vi "Post-Install Custom Action.vi"(10 "Variant":variant) -> (0 "error out":errorcluster)   [LabVIEW 2020]
uses:
  <vilib>/zip/NI_Unzip.lvlib
  <vilib>/ErrorRing/Error Ring.xnode
  <vilib>/Utility/error.llb/Error Cluster From Error Code.vi
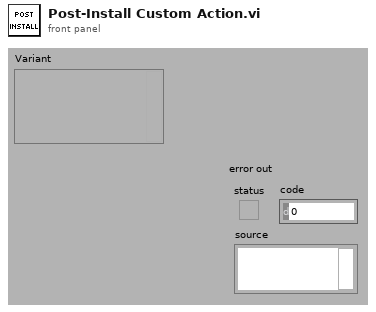
[diagram p1: front panel]
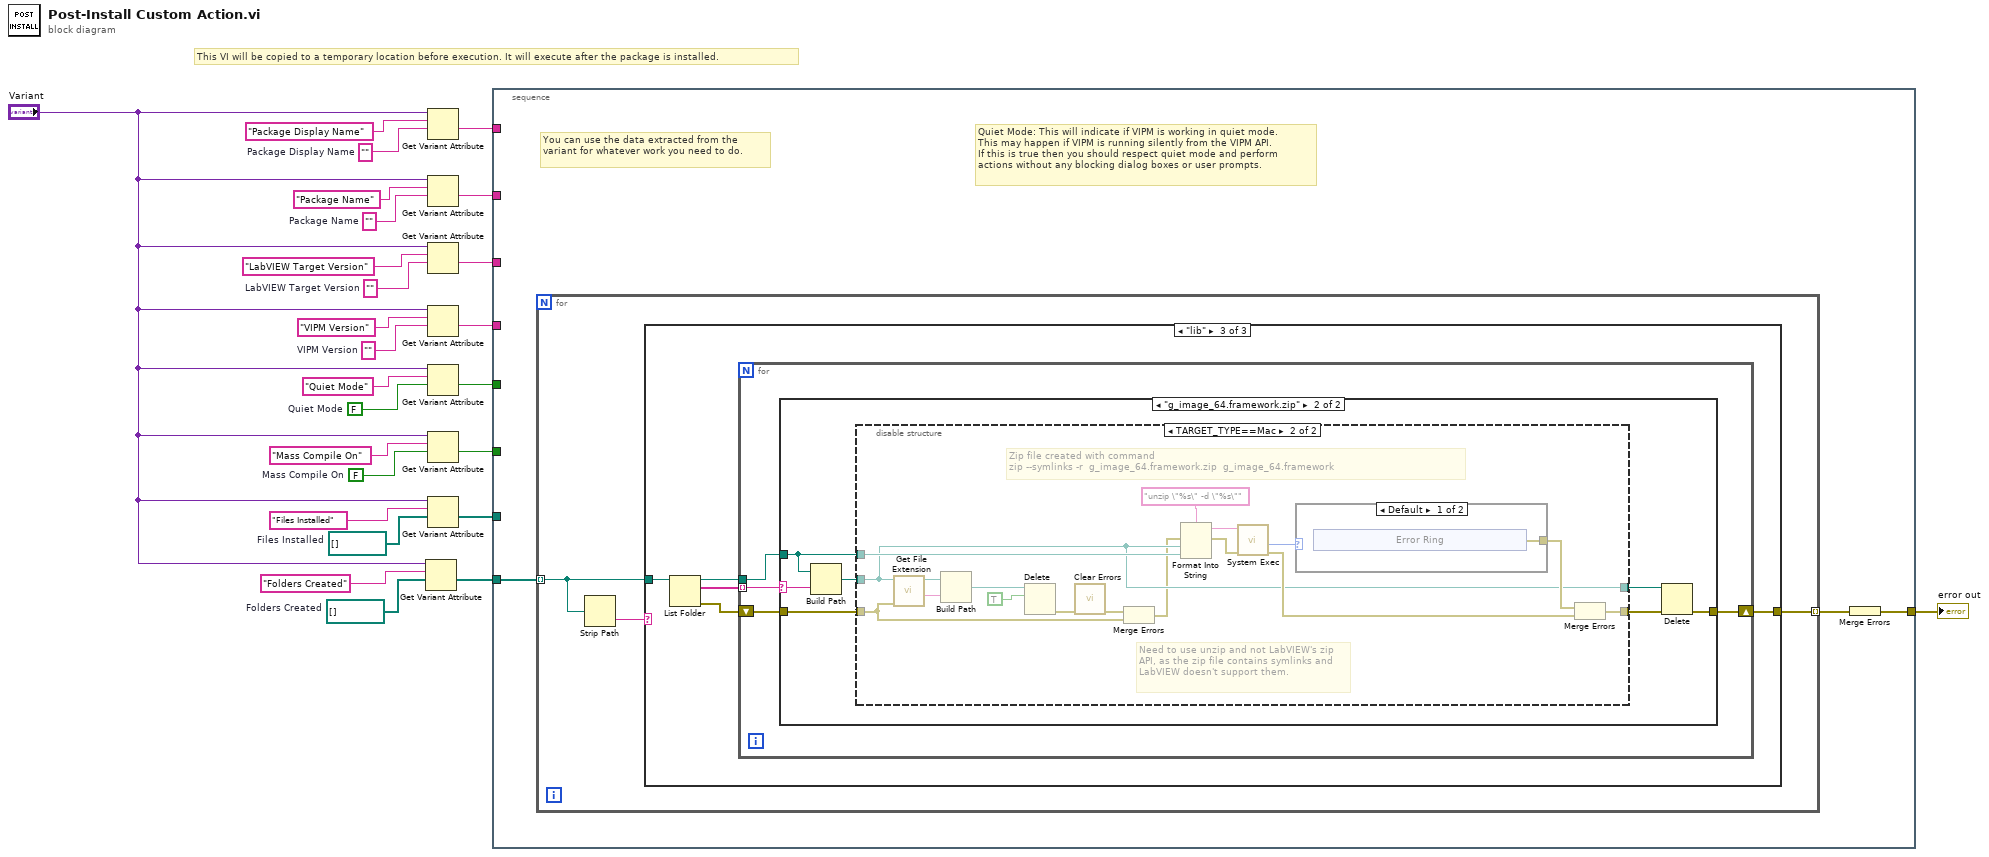
[diagram p0: block diagram]
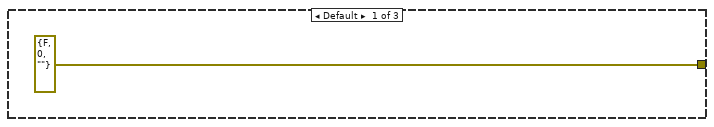
[diagram p2: hidden frame]
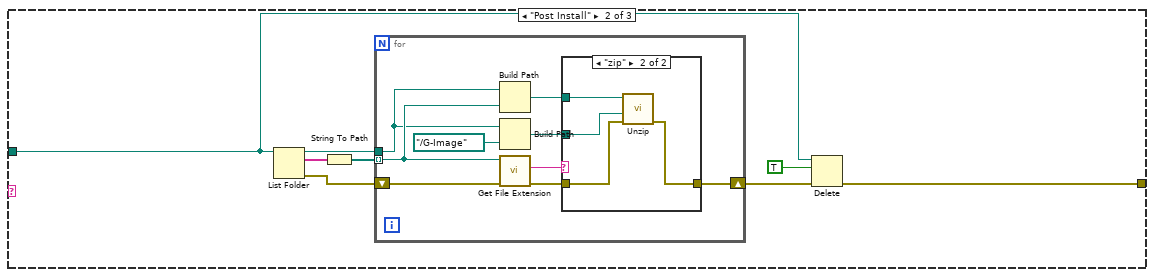
[diagram p3: hidden frame]
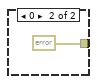
[diagram p7: hidden frame]
diagram:
  w2 = path[] []  # Folders Created
  w3 = path[] []  # Files Installed
  w9 = FALSE  # Mass Compile On
  w10 = ""  # Package Display Name
  w17 = FALSE  # Quiet Mode
  w20 = ""  # VIPM Version
  w22 = ""  # LabVIEW Target Version
  w24 = ""  # Package Name
  # "This VI will be copied to a temporary location before execution. It will execute after the package is installed."
  n1 = Get Variant Attribute(Variant="Variant", name="Folders Created", default value (empty Variant)=w2) -> (value=w7:path[])  [unwired: 1 in, 3 out]
  n2 = Get Variant Attribute(Variant="Variant", name="Package Display Name", default value (empty Variant)=w10) -> (value=w16:string)  [unwired: 1 in, 3 out]
  n3 = Get Variant Attribute(Variant="Variant", name="Package Name", default value (empty Variant)=w24) -> (value=w15:string)  [unwired: 1 in, 3 out]
  n4 = Get Variant Attribute(Variant="Variant", name="LabVIEW Target Version", default value (empty Variant)=w22) -> (value=w14:string)  [unwired: 1 in, 3 out]
  n5 = Get Variant Attribute(Variant="Variant", name="VIPM Version", default value (empty Variant)=w20) -> (value=w13:string)  [unwired: 1 in, 3 out]
  n6 = Get Variant Attribute(Variant="Variant", name="Quiet Mode", default value (empty Variant)=w17) -> (value=w12:bool)  [unwired: 1 in, 3 out]
  n7 = Get Variant Attribute(Variant="Variant", name="Mass Compile On", default value (empty Variant)=w9) -> (value=w11:bool)  [unwired: 1 in, 3 out]
  n8 = Get Variant Attribute(Variant="Variant", name="Files Installed", default value (empty Variant)=w3) -> (value=w6:path[])  [unwired: 1 in, 3 out]
  n9 = stacked-sequence {
    tunnel: w16 -> [_]
    tunnel: w15 -> [_]
    tunnel: w14 -> [_]
    tunnel: w13 -> [_]
    tunnel: w12 -> [_]
    tunnel: w11 -> [_]
    tunnel: w6 -> [_]
    tunnel: w7 -> [w29]
    tunnel: [w27] -> w1
    frame #0 {
      # "Quiet Mode: This will indicate if VIPM is working in quiet mode.\nThis may happen if VIPM is running silently from the VIPM API.\nIf this is true then you should respect quiet mode and perform\nactions without any blocking dialog boxes or user prompts."
      # "You can use the data extracted from the variant for whatever work you need to do."
      n10 = for {
        tunnel: w29 -> [w32] mode=indexing
        tunnel: [w31] -> w28 mode=indexing
        n11 = Strip Path(path=w32) -> (name=w30:string)  [unwired: 1 out]
        n12 = case shown="\"lib\"" w30 {
          tunnel: w32 -> [_ w35 w58]
          tunnel: [errorcluster {"status"=FALSE, "code"=0, "source"=""} ("error out") w36 w57] -> w31
          frame Default {
          }
          frame "Post Install" {
            n13 = List Folder(path=w35) -> (path out=w39:path, filenames=w41:string[], error out=w38:errorcluster)  [unwired: 3 in, 1 out]
            n14 = String To Path(string=w41) -> (path=w40:path[])
            n15 = for {
              tunnel: w40 -> [w50] mode=indexing
              tunnel: w39 -> [w43]
              shift-right: [w45] -> w37
              shift-left: w38 -> [w47]
              n16 = Build Path(base path=w43, name or relative path=w50) -> (appended path=w48:path)
              n17 = Build Path(base path=w43, name or relative path=path "../G-Image" ("Target directory (same as Zip file if empty)")) -> (appended path=w42:path)
              n18 = call <vilib>:"Get File Extension.vi"("error in (no error)"=w47, "file"=w50) -> ("error out"=w46:errorcluster, "lowercase file extension"=w49:string)  [unwired: 5 in, 3 out]
              n19 = case shown="\"zip\"" w49 {
                tunnel: w48 -> [_ w55]
                tunnel: w46 -> [w51 w54]
                tunnel: [w51 w53] -> w45
                tunnel: w42 -> [_ w52]
                frame Default {
                }
                frame "zip" {
                  n20 = call <vilib>:"Unzip.vi"("error in (no error)"=w54, "Target directory (same as Zip file if empty)"=w52, "Zip file"=w55) -> ("error out"=w53:errorcluster)  [unwired: 6 in, 2 out]
                }
              }
            }
            n21 = Delete(path (use dialog)=w35, entire hierarchy (F)=TRUE, error in=w37) -> (error out=w36:errorcluster)  [unwired: 2 in, 2 out]
          }
          frame "lib" {
            n22 = List Folder(path=w58) -> (path out=w60:path, filenames=w56:string[], error out=w59:errorcluster)  [unwired: 3 in, 1 out]
            n23 = for {
              tunnel: w60 -> [w61]
              shift-right: [w64] -> w57
              shift-left: w59 -> [w63]
              tunnel: w56 -> [w62] mode=indexing
              n24 = case shown="\"g_image_64.framework.zip\"" w62 {
                selector: w62 -> [_ w72]
                tunnel: w63 -> [w65 w70]
                tunnel: [w65 w68] -> w64
                tunnel: w61 -> [_ w67]
                frame Default {
                }
                frame "g_image_64.framework.zip" {
                  n25 = Build Path(base path=w67, name or relative path=w72) -> (appended path=w71:path)
                  n26 = disable-structure shown="TARGET_TYPE==Mac" {
                    disable-tunnel: w71 -> [w73 w81]
                    disable-tunnel: w67 -> [_ w89]
                    disable-tunnel: w70 -> [w74 w77]
                    disable-tunnel: [w74 w87] -> w69
                    disable-tunnel: [w73 w81] -> w66
                    frame condition #0 (active) {
                    }
                    frame condition #1 {
                      # "Zip file created with command\nzip --symlinks -r  g_image_64.framework.zip  g_image_64.framework"
                      # "Need to use unzip and not LabVIEW's zip API, as the zip file contains symlinks and LabVIEW doesn't support them."
                      n27 = call <vilib>:"Get File Extension.vi"("error in (no error)"=w77, "file"=w81) -> ("filename without extension"=w82:string, "dup file"=w79:path)  [unwired: 5 in, 3 out]
                      n28 = Build Path(base path=w79, name or relative path=w82) -> (appended path=w80:path)
                      n29 = Delete(path (use dialog)=w80, entire hierarchy (F)=TRUE) -> (error out=w78:errorcluster)  [unwired: 3 in, 2 out]
                      n30 = call <vilib>:"Clear Errors.vi"("error in (no error)"=w78) -> ("error out"=w76:errorcluster)  [unwired: 5 in, 1 out]
                      n31 = Merge Errors(w76, w77) -> (w75:errorcluster)
                      n32 = Format Into String(format string="unzip \"%s\" -d \"%s\"" ("command line"), error in=w75, w81, w89) -> (resulting string=w86:string, error out=w90:errorcluster)  [unwired: 1 in]
                      n33 = call <vilib>:"System Exec.vi"("error in (no error)"=w90, "command line"=w86) -> ("error out"=w84:errorcluster, "return code"=w85:i32)  [unwired: 6 in, 2 out]
                      n34 = case shown="Default" w85 {
                        tunnel: [w92 errorcluster {"status"=FALSE, "code"=0, "source"=""} ("error out")] -> w88
                        frame Default {
                          n35 = xnode "Error Ring"() -> ("error out"=w92:errorcluster)
                        }
                        frame 0 {
                        }
                      }
                      n36 = Merge Errors(w88, w84) -> (w87:errorcluster)
                    }
                  }
                  n37 = Delete(path (use dialog)=w66, error in=w69) -> (error out=w68:errorcluster)  [unwired: 3 in, 2 out]
                }
              }
            }
          }
        }
      }
      n38 = Merge Errors(w28) -> (w27:errorcluster)
    }
  }
  "error out" <- w1
